vi "Update Model Info.vi"(8 "error in (no error)":errorcluster, 11 "Loop Data":T1) -> (0 "error out":errorcluster)   [LabVIEW 2016, in "System Mapping Tool.lvlib"]
uses:
  System Mapping Tool.lvlib
  TypeDefs/Model Analysis Data.ctl
  TypeDefs/Model Analysis UI Refs.ctl
  NationalInstruments.VeriStand.SystemStorageUI
  NationalInstruments.VeriStand.SystemDefinitionAPI
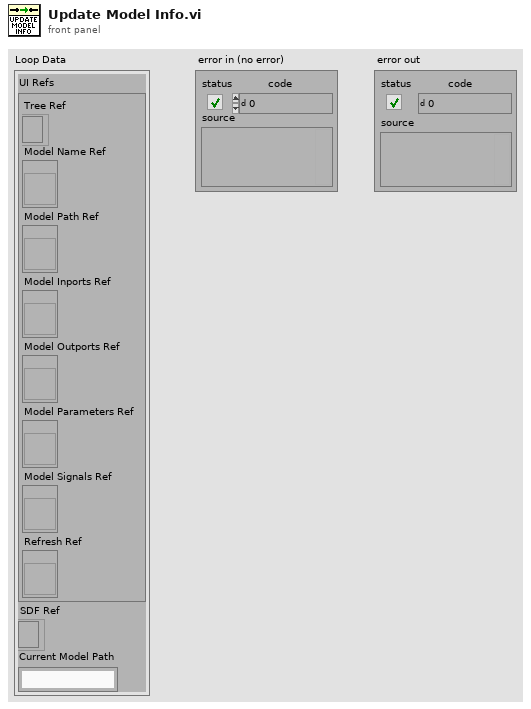
[diagram p1: front panel]
types:
  T1 = typedef "System Mapping Tool.lvlib/Model Analysis Data.ctl" = cluster{"UI Refs":T2, "SDF Ref":refnum<k24>, "Current Model Path":string}
  T2 = typedef "System Mapping Tool.lvlib/Model Analysis UI Refs.ctl" = cluster{"Tree Ref":refnum<k24>, "Model Name Ref":refnum<vi>, "Model Path Ref":refnum<vi>, "Model Inports Ref":refnum<vi>, "Model Outports Ref":refnum<vi>, "Model Parameters Ref":refnum<vi>, "Model Signals Ref":refnum<vi>, "Refresh Ref":refnum<vi>}
  T3 = enum8{"Enabled", "Disabled", "Disabled and Grayed Out"}
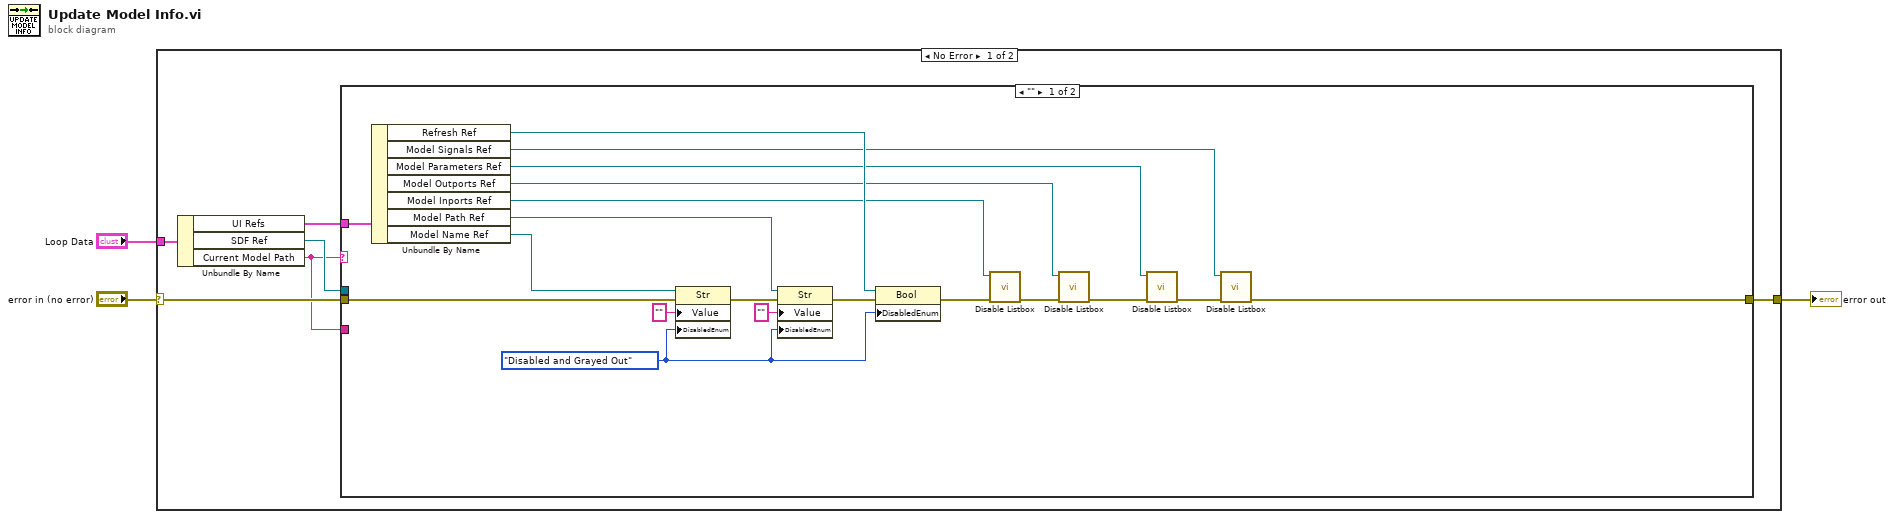
[diagram p0: block diagram]
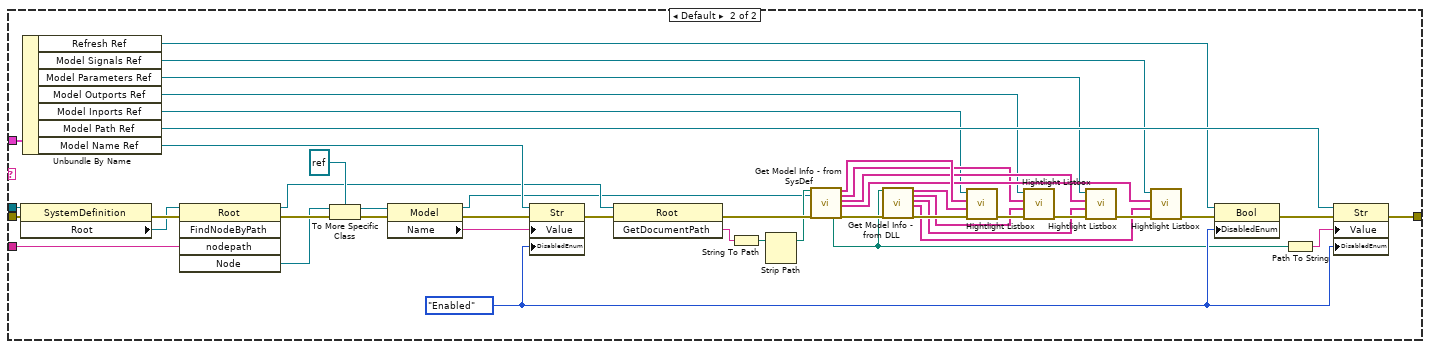
[diagram p2: hidden frame]
diagram:
  n1 = case shown="No Error" "error in (no error)" {
    selector: "error in (no error)" -> [w8 w75]
    tunnel: [w5 w75] -> w2
    tunnel: "Loop Data" -> [w9 _]
    frame No Error {
      n2 = Unbundle By Name(w9) -> ("UI Refs"=w4:T2, "SDF Ref"=w7:refnum<k24>, "Current Model Path"=w6:string)
      n3 = case shown="\"\"" w6 {
        tunnel: w8 -> [w27 w74]
        tunnel: w7 -> [_ w59]
        tunnel: w6 -> [_ w72]
        tunnel: [w14 w31] -> w5
        tunnel: w4 -> [w26 w66]
        frame "" {
          w20 = T3."Disabled and Grayed Out" ("Disabled")
          n4 = Unbundle By Name(w26) -> ("Refresh Ref"=w21:refnum<vi>, "Model Signals Ref"=w13:refnum<vi>, "Model Parameters Ref"=w12:refnum<vi>, "Model Outports Ref"=w11:refnum<vi>, "Model Inports Ref"=w10:refnum<vi>, "Model Path Ref"=w22:refnum<vi>, "Model Name Ref"=w25:refnum<vi>)
          n5 = property class="Str"(reference=w25, error in=w27, "Value"="", "DisabledEnum"=w20) -> (error out=w28:errorcluster)  [unwired: 1 out]
          n6 = property class="Str"(reference=w22, error in=w28, "Value"="", "DisabledEnum"=w20) -> (error out=w19:errorcluster)  [unwired: 1 out]
          n7 = property class="Bool"(reference=w21, error in=w19, "DisabledEnum"=w20) -> (error out=w18:errorcluster)  [unwired: 1 out]
          n8 = call "Disable Listbox.vi"("error in (no error)"=w18, "Listbox Ref"=w10) -> ("error out"=w17:errorcluster)  [unwired: 9 in]
          n9 = call "Disable Listbox.vi"("error in (no error)"=w17, "Listbox Ref"=w11) -> ("error out"=w16:errorcluster)  [unwired: 9 in]
          n10 = call "Disable Listbox.vi"("error in (no error)"=w16, "Listbox Ref"=w12) -> ("error out"=w15:errorcluster)  [unwired: 9 in]
          n11 = call "Disable Listbox.vi"("error in (no error)"=w15, "Listbox Ref"=w13) -> ("error out"=w14:errorcluster)  [unwired: 9 in]
        }
        frame Default {
          w61 = T3."Enabled" ("Disabled")
          n12 = property class="SystemDefinition"(reference=w59, error in=w74) -> (error out=w73:errorcluster, "Root"=w58:refnum<k24>)  [unwired: 1 out]
          n13 = Unbundle By Name(w66) -> ("Refresh Ref"=w62:refnum<vi>, "Model Signals Ref"=w35:refnum<vi>, "Model Parameters Ref"=w36:refnum<vi>, "Model Outports Ref"=w37:refnum<vi>, "Model Inports Ref"=w38:refnum<vi>, "Model Path Ref"=w63:refnum<vi>, "Model Name Ref"=w65:refnum<vi>)
          n14 = invoke class="Root" method="FindNodeByPath"(reference=w58, error in=w73, "nodepath"=w72) -> (reference out=w55:refnum<k24>, error out=w71:errorcluster, "Node"=w70:refnum<k24>)  [unwired: 2 in, 2 out]
          n15 = To More Specific Class(target class=refnum<k24> refnum (".NET object"), reference=w70, error in=w71) -> (specific class reference=w69:refnum<k24>, error out=w60:errorcluster)
          n16 = property class="Model"(reference=w69, error in=w60) -> (reference out=w52:refnum<k24>, error out=w67:errorcluster, "Name"=w64:string)
          n17 = property class="Str"(reference=w65, error in=w67, "Value"=w64, "DisabledEnum"=w61) -> (error out=w33:errorcluster)  [unwired: 1 out]
          n18 = invoke class="Root" method="GetDocumentPath"(reference=w55, error in=w33) -> (error out=w54:errorcluster, "GetDocumentPath"=w56:string)  [unwired: 1 in, 1 out]
          n19 = String To Path(string=w56) -> (path=w57:path)
          n20 = Strip Path(path=w57) -> (stripped path=w53:path)  [unwired: 1 out]
          n21 = call "Get Model Info - from SysDef.vi"("System Definition Filepath (.nivssdf)"=w53, "Model Ref"=w52, "Error (in)"=w54) -> ("Model Path"=w30:path, "SysDef Inports"=w46:string[], "SysDef Outports"=w39:string[], "SysDef Parameters"=w42:string[], "SysDef Signals"=w43:string[], "Error (out)"=w51:errorcluster)  [unwired: 10 in, 1 out]
          n22 = call "Get Model Info - from DLL.vi"("Model Filepath"=w30, "Error (in)"=w51) -> ("DLL Inports"=w45:string[], "DLL Outports"=w40:string[], "DLL Parameters"=w41:string[], "DLL Signals"=w44:string[], "Error (out)"=w50:errorcluster)  [unwired: 13 in]
          n23 = call "Hightlight Listbox.vi"("error in (no error)"=w50, "From DLL"=w45, "From SDF"=w46, "Listbox Ref"=w38) -> ("error out"=w49:errorcluster)  [unwired: 7 in]
          n24 = call "Hightlight Listbox.vi"("error in (no error)"=w49, "From DLL"=w40, "From SDF"=w39, "Listbox Ref"=w37) -> ("error out"=w48:errorcluster)  [unwired: 7 in]
          n25 = call "Hightlight Listbox.vi"("error in (no error)"=w48, "From DLL"=w41, "From SDF"=w42, "Listbox Ref"=w36) -> ("error out"=w47:errorcluster)  [unwired: 7 in]
          n26 = call "Hightlight Listbox.vi"("error in (no error)"=w47, "From DLL"=w44, "From SDF"=w43, "Listbox Ref"=w35) -> ("error out"=w34:errorcluster)  [unwired: 7 in]
          n27 = property class="Bool"(reference=w62, error in=w34, "DisabledEnum"=w61) -> (error out=w32:errorcluster)  [unwired: 1 out]
          n28 = Path To String(path=w30) -> (string=w29:string)
          n29 = property class="Str"(reference=w63, error in=w32, "Value"=w29, "DisabledEnum"=w61) -> (error out=w31:errorcluster)  [unwired: 1 out]
        }
      }
    }
    frame Error {
    }
  }
  "error out" <- w2
